vi "collect_data.vi"(6 "data?":bool, 7 "Resolution":u32=200, 8 "error in (no error)":errorcluster, 9 "progress":refnum<vi>, 10 "No. of values":i32=100, 11 "handle":i32) -> (0 "error out":errorcluster, 3 "Dataset":T1(array[cluster]))   [LabVIEW 2018]
uses:
  <userlib>/Gigahertz-Optik/GOMDTR9600/GOMDTR9600.lvlib
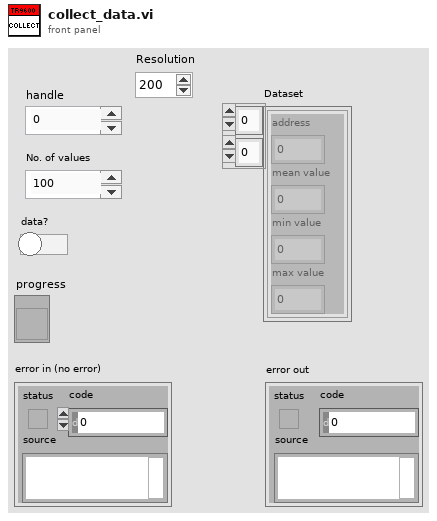
[diagram p1: front panel]
types:
  T1 = cluster{"address":i32, "mean value":dbl, "min value":dbl, "max value":dbl}[][]
  T2 = cluster{"address":i32, "mean value":dbl, "min value":dbl, "max value":dbl}[]
  T3 = cluster{"address":i32, "mean value":dbl, "min value":dbl, "max value":dbl}
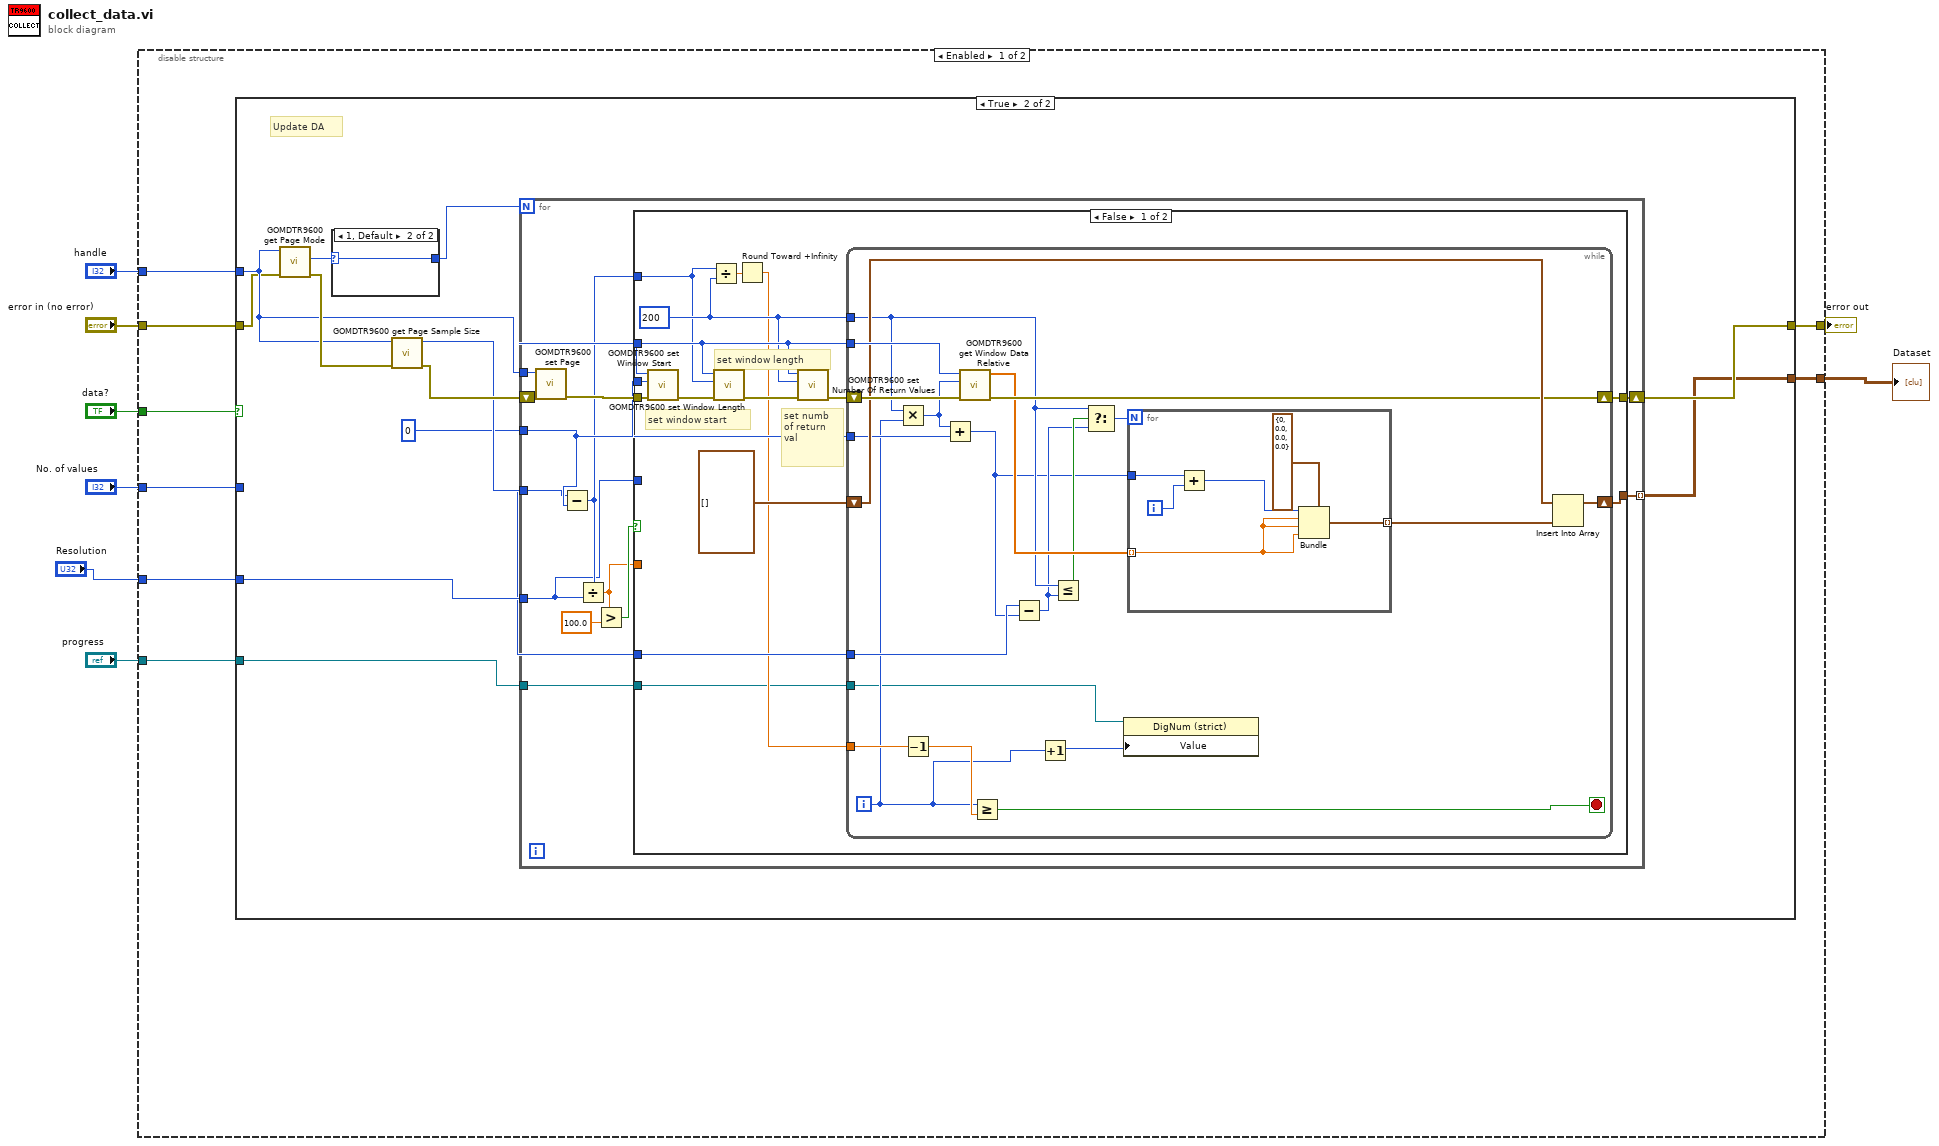
[diagram p0: block diagram]
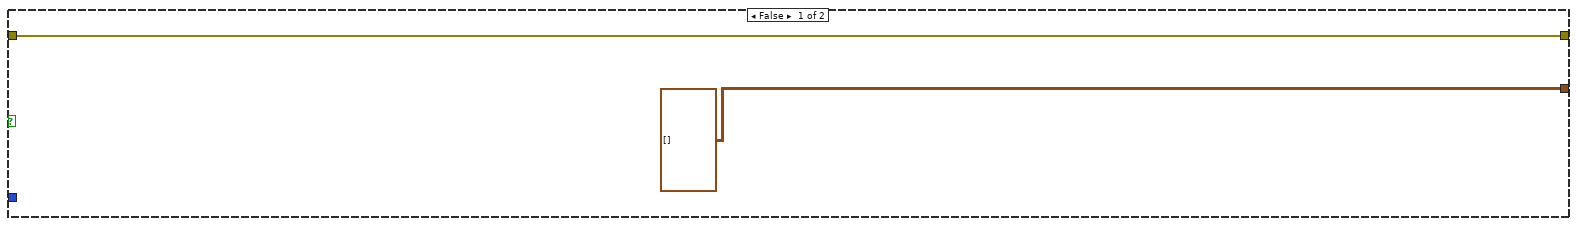
[diagram p2: hidden frame]
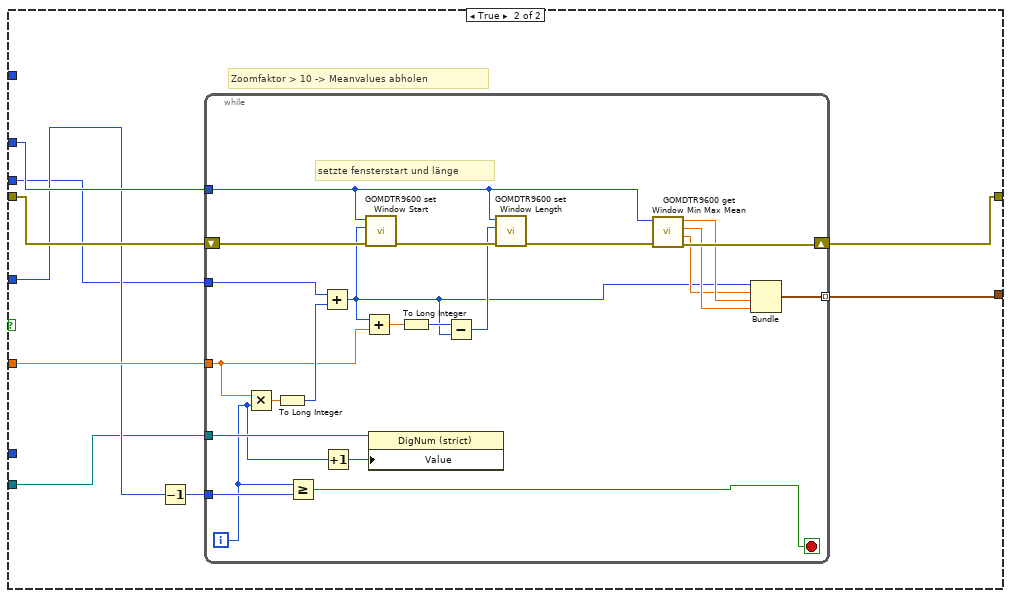
[diagram p3: hidden frame]
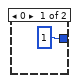
[diagram p4: hidden frame]
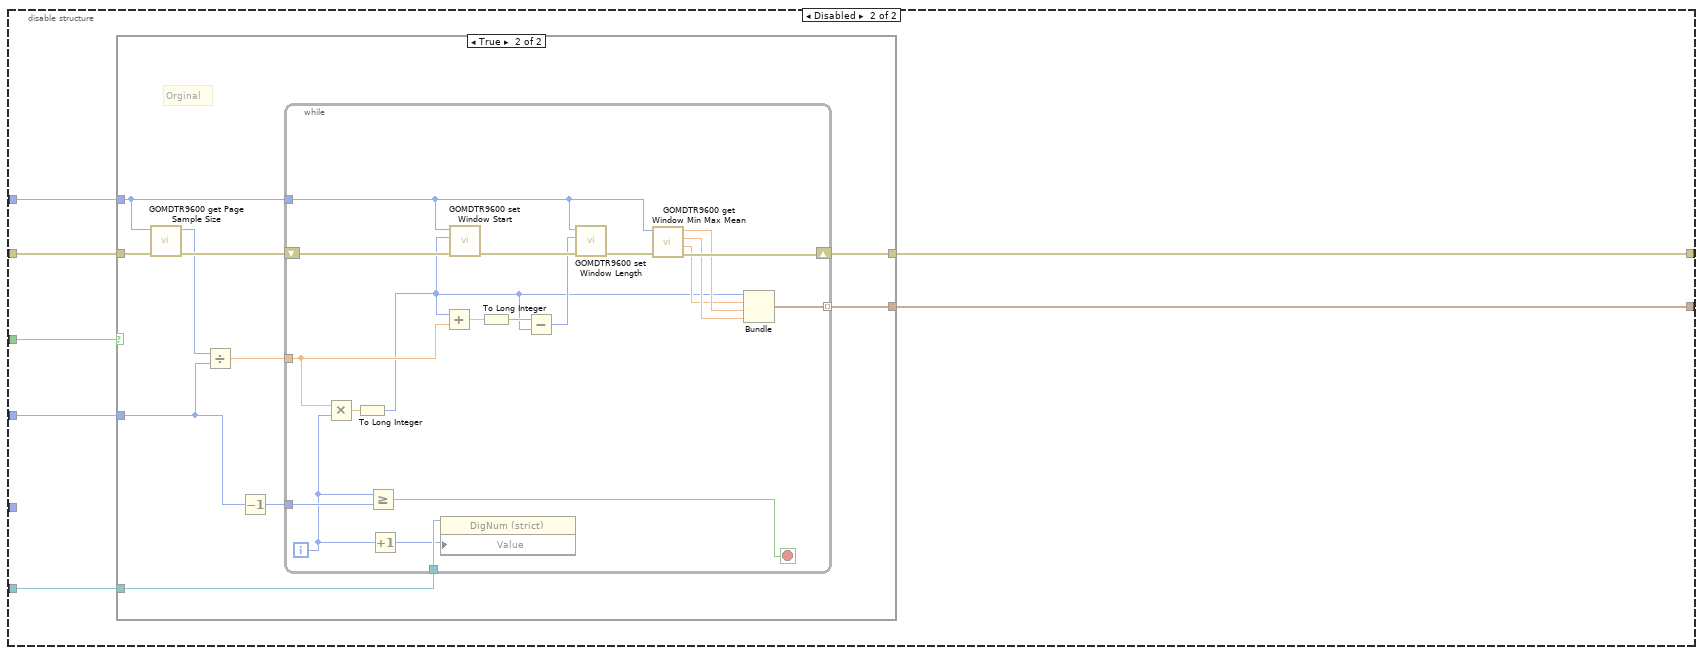
[diagram p5: hidden frame]
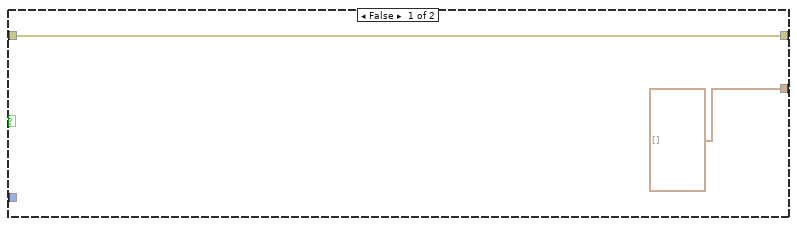
[diagram p6: hidden frame]
diagram:
  n1 = disable-structure shown="Enabled" {
    disable-tunnel: [w16 w125] -> w8
    disable-tunnel: "data?" -> [w15 w124]
    disable-tunnel: [w14 w123] -> w6
    disable-tunnel: "handle" -> [w13 w122]
    disable-tunnel: "error in (no error)" -> [w12 w121]
    disable-tunnel: "progress" -> [w11 w120]
    disable-tunnel: "No. of values" -> [w10 w119]
    disable-tunnel: "Resolution" -> [w9 _]
    frame Enabled {
      n2 = case shown="True" w15 {
        tunnel: [w18 w21] -> w16
        tunnel: [T1 [] w20] -> w14
        tunnel: w12 -> [w18 w23]
        tunnel: w13 -> [_ w24]
        tunnel: w11 -> [_ w22]
        tunnel: w10 -> [_ _]
        tunnel: w9 -> [_ w19]
        frame False {
        }
        frame True {
          # "Update DA"
          n3 = call <userlib>:"GOMDTR9600 get Page Mode.vi"("error in (no error)"=w23, "handle"=w24) -> ("error out"=w29:errorcluster, "value"=w26:i32)  [unwired: 7 in, 1 out]
          n4 = case shown="1, Default" w26 {
            selector: w26 -> [_ w118]
            tunnel: [1 ("#ofpages") w118] -> w28
            frame 0 {
            }
            frame 1, Default {
            }
          }
          n5 = call <userlib>:"GOMDTR9600 get Page Sample Size.vi"("error in (no error)"=w29, "handle"=w24) -> ("error out"=w30:errorcluster, "value"=w27:i32)  [unwired: 7 in, 1 out]
          n6 = for {
            N: w28 -> [_]
            tunnel: 0 ("start adress") -> [w42]
            tunnel: w24 -> [w41]
            tunnel: w27 -> [w40]
            shift-right: [w38] -> w21
            shift-left: w30 -> [w39]
            tunnel: w22 -> [w37]
            tunnel: [w36] -> w20 mode=indexing
            tunnel: w19 -> [w31]
            n7 = call <userlib>:"GOMDTR9600 set Page.vi"("error in (no error)"=w39, "handle"=w41) -> ("error out"=w43:errorcluster)  [unwired: 8 in, 1 out]
            n8 = Subtract(x=w40, y=w42) -> (x-y=w35:i32)
            n9 = Divide(x=w35, y=w31) -> (x/y=w32:dbl)
            n10 = Greater?(x=w32, y=100.0) -> (0:w33:bool)
            n11 = case shown="False" w33 {
              tunnel: w43 -> [w58 w93]
              tunnel: w42 -> [w57 w89]
              tunnel: w41 -> [w56 w92]
              tunnel: w40 -> [w55 _]
              tunnel: [w47 w87] -> w38
              tunnel: w37 -> [w46 w88]
              tunnel: [w45 w86] -> w36
              tunnel: w35 -> [w44 _]
              tunnel: w32 -> [_ w91]
              tunnel: w31 -> [_ w90]
              frame False {
                w49 = 200 ("value")
                # "set numb\nof return \nval"
                # "set window length"
                # "set window start"
                n12 = call <userlib>:"GOMDTR9600 set Window Start.vi"("error in (no error)"=w58, "value"=w57, "handle"=w56) -> ("error out"=w53:errorcluster)  [unwired: 7 in, 1 out]
                n13 = Divide(x=w44, y=w49) -> (x/y=w50:dbl)
                n14 = call <userlib>:"GOMDTR9600 set Window Length.vi"("error in (no error)"=w53, "value"=w44, "handle"=w56) -> ("error out"=w52:errorcluster)  [unwired: 7 in, 1 out]
                n15 = Round Toward +Infinity(x=w50) -> (ceil(x): smallest int >= x=w48:dbl)
                n16 = call <userlib>:"GOMDTR9600 set Number Of Return Values.vi"("error in (no error)"=w52, "value"=w49, "handle"=w56) -> ("error out"=w54:errorcluster)  [unwired: 7 in, 1 out]
                n17 = while {
                  tunnel: w56 -> [w78]
                  shift-right: [w75] -> w47
                  shift-left: w54 -> [w79]
                  shift-right: [w76] -> w45
                  shift-left: T2 [] -> [w77]
                  tunnel: w49 -> [w68]
                  tunnel: w57 -> [w74]
                  tunnel: w48 -> [w73]
                  tunnel: w55 -> [w70]
                  tunnel: w46 -> [w59]
                  i -> [w60]
                  stop <- w62 stop-if-true
                  n18 = Multiply(x=w68, y=w60) -> (x*y=w63:i32)
                  n19 = Decrement(x=w73) -> (x-1=w72:dbl)
                  n20 = Add(x=w63, y=w74) -> (x+y=w64:i32)
                  n21 = call <userlib>:"GOMDTR9600 get Window Data Relative.vi"("error in (no error)"=w79, "sampleNumber"=w63, "handle"=w78) -> ("error out"=w75:errorcluster, "value"=w71:dbl[])  [unwired: 6 in, 1 out]
                  n22 = Greater Or Equal?(x=w60, y=w72) -> (x >= y?=w62:bool)
                  n23 = Subtract(x=w70, y=w64) -> (x-y=w67:i32)
                  n24 = Increment(x=w60) -> (x+1=w61:i32)
                  n25 = Less Or Equal?(x=w68, y=w67) -> (x <= y?=w69:bool)
                  n26 = Select(t=w68, s=w69, f=w67) -> (s? t:f=w66:i32)
                  n27 = property class="DigNum (strict)"(reference=w59, "Value"=w61) -> ()  [unwired: 1 in, 2 out]
                  n28 = for {
                    N: w66 -> [_]
                    tunnel: w64 -> [w85]
                    tunnel: w71 -> [w80] mode=indexing
                    tunnel: [w82] -> w65 mode=indexing
                    i -> [w84]
                    n29 = Add(x=w85, y=w84) -> (x+y=w83:i32)
                    n30 = Bundle(cluster=T3 {"address"=0, "mean value"=0.0, "min value"=0.0, "max value"=0.0} ("output cluster"), "address"=w83, "mean value"=w80, "min value"=w80, "max value"=w80) -> (w82:T3)
                  }
                  n31 = Insert Into Array(array=w77, new element=w65) -> (w76:T2)  [unwired: 1 in]
                }
              }
              frame True {
                # "Zoomfaktor > 10 -> Meanvalues abholen"
                n32 = Decrement(x=w90) -> (x-1=w94:u32)
                n33 = while {
                  tunnel: w92 -> [w104]
                  tunnel: [w116] -> w86 mode=indexing
                  shift-right: [w105] -> w87
                  shift-left: w93 -> [w115]
                  tunnel: w91 -> [w107]
                  tunnel: w89 -> [w112]
                  tunnel: w94 -> [w100]
                  tunnel: w88 -> [w98]
                  i -> [w97]
                  stop <- w95 stop-if-true
                  # "setzte fensterstart und länge"
                  n34 = Multiply(x=w107, y=w97) -> (x*y=w113:dbl)
                  n35 = To Long Integer(number=w113) -> (32bit integer=w111:i32)
                  n36 = Greater Or Equal?(x=w97, y=w100) -> (x >= y?=w95:bool)
                  n37 = Add(x=w112, y=w111) -> (x+y=w99:i32)
                  n38 = Increment(x=w97) -> (x+1=w96:i32)
                  n39 = Add(x=w99, y=w107) -> (x+y=w110:dbl)
                  n40 = call <userlib>:"GOMDTR9600 set Window Start.vi"("error in (no error)"=w115, "value"=w99, "handle"=w104) -> ("error out"=w114:errorcluster)  [unwired: 7 in, 1 out]
                  n41 = property class="DigNum (strict)"(reference=w98, "Value"=w96) -> ()  [unwired: 1 in, 2 out]
                  n42 = To Long Integer(number=w110) -> (32bit integer=w109:i32)
                  n43 = Subtract(x=w109, y=w99) -> (x-y=w108:i32)
                  n44 = call <userlib>:"GOMDTR9600 set Window Length.vi"("error in (no error)"=w114, "value"=w108, "handle"=w104) -> ("error out"=w106:errorcluster)  [unwired: 7 in, 1 out]
                  n45 = call <userlib>:"GOMDTR9600 get Window Min Max Mean.vi"("error in (no error)"=w106, "handle"=w104) -> ("error out"=w105:errorcluster, "mean"=w101:dbl, "max"=w102:dbl, "min"=w103:dbl)  [unwired: 5 in, 1 out]
                  n46 = Bundle(w99, "mean"=w101, "min"=w103, "max"=w102) -> (w116:cluster{i32, "mean":dbl, "min":dbl, "max":dbl})  [unwired: 1 in]
                }
              }
            }
          }
        }
      }
    }
    frame Disabled {
      n47 = case shown="True" w124 {
        tunnel: [w127 w137] -> w125
        tunnel: [T2 [] w136] -> w123
        tunnel: w121 -> [w127 w133]
        tunnel: w122 -> [_ w131]
        tunnel: w120 -> [_ w129]
        tunnel: w119 -> [_ w128]
        frame False {
        }
        frame True {
          # "Orginal"
          n48 = call <userlib>:"GOMDTR9600 get Page Sample Size.vi"("error in (no error)"=w133, "handle"=w131) -> ("error out"=w132:errorcluster, "value"=w130:i32)  [unwired: 7 in, 1 out]
          n49 = Divide(x=w130, y=w128) -> (x/y=w135:dbl)
          n50 = Decrement(x=w128) -> (x-1=w134:i32)
          n51 = while {
            tunnel: w131 -> [w147]
            tunnel: [w157] -> w136 mode=indexing
            shift-right: [w148] -> w137
            shift-left: w132 -> [w156]
            tunnel: w135 -> [w150]
            tunnel: w134 -> [w143]
            tunnel: w129 -> [w140]
            i -> [w139]
            stop <- w142 stop-if-true
            n52 = Multiply(x=w150, y=w139) -> (x*y=w154:dbl)
            n53 = To Long Integer(number=w154) -> (32bit integer=w141:i32)
            n54 = Greater Or Equal?(x=w139, y=w143) -> (x >= y?=w142:bool)
            n55 = Increment(x=w139) -> (x+1=w138:i32)
            n56 = property class="DigNum (strict)"(reference=w140, "Value"=w138) -> ()  [unwired: 1 in, 2 out]
            n57 = Add(x=w141, y=w150) -> (x+y=w153:dbl)
            n58 = call <userlib>:"GOMDTR9600 set Window Start.vi"("error in (no error)"=w156, "value"=w141, "handle"=w147) -> ("error out"=w155:errorcluster)  [unwired: 7 in, 1 out]
            n59 = To Long Integer(number=w153) -> (32bit integer=w152:i32)
            n60 = Subtract(x=w152, y=w141) -> (x-y=w151:i32)
            n61 = call <userlib>:"GOMDTR9600 set Window Length.vi"("error in (no error)"=w155, "value"=w151, "handle"=w147) -> ("error out"=w149:errorcluster)  [unwired: 7 in, 1 out]
            n62 = call <userlib>:"GOMDTR9600 get Window Min Max Mean.vi"("error in (no error)"=w149, "handle"=w147) -> ("error out"=w148:errorcluster, "mean"=w144:dbl, "max"=w145:dbl, "min"=w146:dbl)  [unwired: 5 in, 1 out]
            n63 = Bundle(w141, "mean"=w144, "min"=w146, "max"=w145) -> (w157:cluster{i32, "mean":dbl, "min":dbl, "max":dbl})  [unwired: 1 in]
          }
        }
      }
    }
  }
  "error out" <- w8
  "Dataset" <- w6
